vi "PWA fire and acquire TOF.vi"() -> (0 "Cumulative Error":errorcluster, 1 "External mode":bool, 2 "Base 10 TOF (signed, \nmu.sec) (I16)":i16)   [LabVIEW 2010]
uses:
  <vilib>/DAQmx/write.llb/DAQmx Write (Digital Bool 1Line 1Point).vi
  <vilib>/DAQmx/read.llb/DAQmx Read (Digital Bool 1Line 1Point).vi
  <vilib>/DAQmx/read.llb/DAQmx Read (Digital 1D Bool NChan 1Samp 1Line).vi
  PWAtasksGLOBAL.vi
  <vilib>/daqmx/miscellaneous.llb/DAQmx Fill In Error Info.vi
panel:
  out "Read High":errorcluster
  out "Switch High":errorcluster
  out "Read Low":errorcluster
  out "Switch Low":errorcluster
  out "Wait":errorcluster
  out "Fire":errorcluster
  out "Sign bit\n(green +, red -)":bool
  out "Base 8 TOF (unsigned)":string="0000"
  out "Low bits":u32
  out "High bits":u32
  out "High bits 7 to 11 (LSB on right)":bool[](array[boolean])
  out "Low bits 0 to 6 (LSB on right)":bool[](array[boolean])
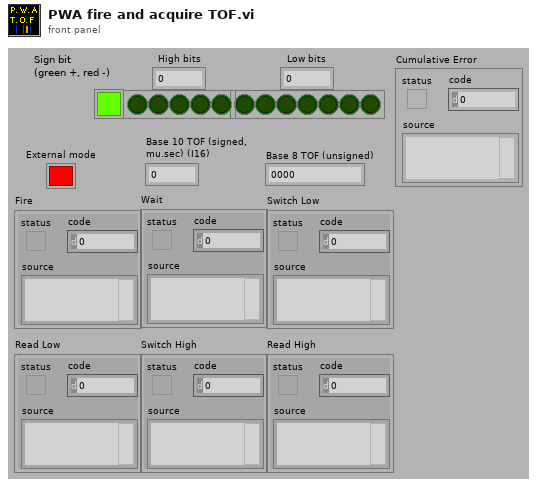
[diagram p1: front panel]
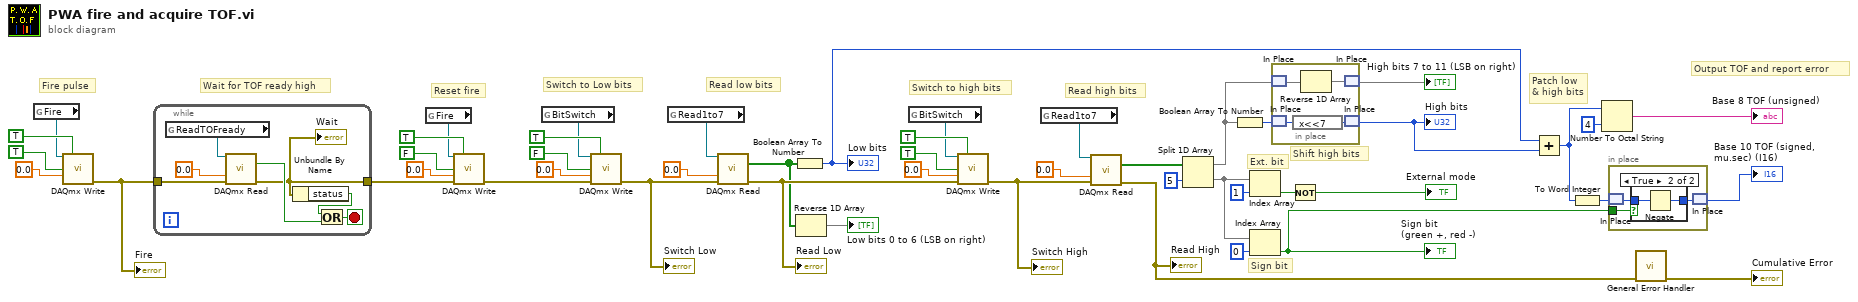
[diagram p0: block diagram]
diagram:
  # "Patch low & high bits"
  # "Output TOF and report error"
  # "Reset fire"
  # "Shift high bits"
  # "Ext. bit"
  # "Sign bit"
  # "Read high bits"
  # "Switch to high bits"
  # "Read low bits"
  # "Switch to Low bits"
  # "Wait for TOF ready high"
  # "Fire pulse"
  n1 = global read "PWAtasksGLOBAL.vi" "Fire"() -> (w39:refnum<k21>)
  n2 = call-poly <vilib>:"DAQmx Write.vi"("task/channels in"=w39, "auto start"=TRUE ("data"), "data"=TRUE, "timeout"=0.0) -> ("error out"=w47:errorcluster)  [unwired: 9 in, 2 out]
  "Fire" <- w47
  n3 = while {
    tunnel: w47 -> [w53]
    tunnel: [w49] -> w9
    stop <- w51 stop-if-true
    n4 = global read "PWAtasksGLOBAL.vi" "ReadTOFready"() -> (w54:refnum<k21>)
    n5 = call-poly <vilib>:"DAQmx Read.vi"("task/channels in"=w54, "timeout"=0.0, "error in"=w53) -> ("data"=w52:bool, "error out"=w49:errorcluster)  [unwired: 10 in, 1 out]
    "Wait" <- w49
    n6 = Unbundle By Name(w49) -> ("status"=w50:bool)
    n7 = Or(x=w50, y=w52) -> (x .or. y?=w51:bool)
  }
  n8 = global read "PWAtasksGLOBAL.vi" "Fire"() -> (w14:refnum<k21>)
  n9 = call-poly <vilib>:"DAQmx Write.vi"("task/channels in"=w14, "auto start"=TRUE ("data"), "data"=FALSE, "timeout"=0.0, "error in"=w9) -> ("error out"=w8:errorcluster)  [unwired: 8 in, 2 out]
  n10 = global read "PWAtasksGLOBAL.vi" "BitSwitch"() -> (w35:refnum<k21>)
  n11 = call-poly <vilib>:"DAQmx Write.vi"("task/channels in"=w35, "auto start"=TRUE ("data"), "data"=FALSE, "timeout"=0.0, "error in"=w8) -> ("error out"=w46:errorcluster)  [unwired: 8 in, 2 out]
  "Switch Low" <- w46
  n12 = global read "PWAtasksGLOBAL.vi" "Read1to7"() -> (w31:refnum<k21>)
  n13 = call-poly <vilib>:"DAQmx Read.vi"("task/channels in"=w31, "timeout"=0.0, "error in"=w46) -> ("data"=w32:bool[], "error out"=w45:errorcluster)  [unwired: 10 in, 1 out]
  "Read Low" <- w45
  n14 = Boolean Array To Number(Boolean array=w32) -> (number=w48:u32)
  "Low bits" <- w48
  n15 = Reverse 1D Array(array=w32) -> (reversed array=→"Low bits 0 to 6 (LSB on right)":bool[])
  n16 = global read "PWAtasksGLOBAL.vi" "BitSwitch"() -> (w27:refnum<k21>)
  n17 = call-poly <vilib>:"DAQmx Write.vi"("task/channels in"=w27, "auto start"=TRUE ("data"), "data"=TRUE, "timeout"=0.0, "error in"=w45) -> ("error out"=w44:errorcluster)  [unwired: 8 in, 2 out]
  "Switch High" <- w44
  n18 = global read "PWAtasksGLOBAL.vi" "Read1to7"() -> (w20:refnum<k21>)
  n19 = call-poly <vilib>:"DAQmx Read.vi"("task/channels in"=w20, "timeout"=0.0, "error in"=w44) -> ("data"=w25:bool[], "error out"=w7:errorcluster)  [unwired: 10 in, 1 out]
  "Read High" <- w7
  n20 = Split 1D Array(array=w25, index=5) -> (first subarray=w6:bool[], second subarray=w22:bool[])
  n21 = Boolean Array To Number(Boolean array=w6) -> (number=w2:u32)
  n22 = Index Array(array=w22, index=1) -> (element=w19:bool)
  n23 = Index Array(array=w22, index=0) -> (element=w43:bool)
  "Sign bit\n(green +, red -)" <- w43
  n24 = in-place {
    n25 = in-place-match #1(w6) -> (w59:bool[])
    n26 = in-place-match #2(w2) -> (w57:u32)
    n27 = expression code="x<<7"(w57) -> (w56:u32)
    n28 = Reverse 1D Array(array=w59) -> (reversed array=w58:bool[])
    n29 = in-place-match #1(w58) -> (→"High bits 7 to 11 (LSB on right)":bool[])
    n30 = in-place-match #2(w56) -> (w1:u32)
  }
  "High bits" <- w1
  n31 = Not(x=w19) -> (.not. x?=→"External mode":bool)
  n32 = Add(x=w48, y=w1) -> (x+y=w11:u32)
  n33 = To Word Integer(number=w11) -> (16bit integer=w4:i16)
  n34 = Number To Octal String(1:i16 4 ("width (-)"), 2:w11) -> (0:→"Base 8 TOF (unsigned)":string)
  n35 = in-place {
    in-place-border: w43 -> [w62]
    n36 = in-place-match #3(w4) -> (w61:i16)
    n37 = case shown="True" w62 {
      tunnel: w61 -> [w63 w65]
      tunnel: [w63 w64] -> w60
      frame False {
      }
      frame True {
        n38 = Negate(x=w65) -> (-x=w64:i16)
      }
    }
    n39 = in-place-match #3(w60) -> (→"Base 10 TOF (signed, \nmu.sec) (I16)":i16)
  }
  n40 = call <vilib>:"General Error Handler.vi"("error in (no error)"=w7) -> ("error out"=→"Cumulative Error":errorcluster)  [unwired: 10 in, 4 out]
